vi "Test Unit Camera1.vi"() -> ()   [LabVIEW 2013]
panel:
  out "ErrorOut 2":errorcluster
  out "CameraNumber":i32
  out "Error out":i32
  out "ErrorOut":errorcluster {"code" format="%x"}
  out "Description":T1 {"GeneralCapabilities 2" format="%032b"; "GeneralCapabilities" format="%032b"; "SensorSubtypeDESC" format="%.0x"; "SensorTypeDESC" format="%.0x"}
  in  "Interface Type":u32=3
  in  "CamNumIn":i32
  in  "Handle in":u64
  out "Error":i32
  out "CameraType":T2
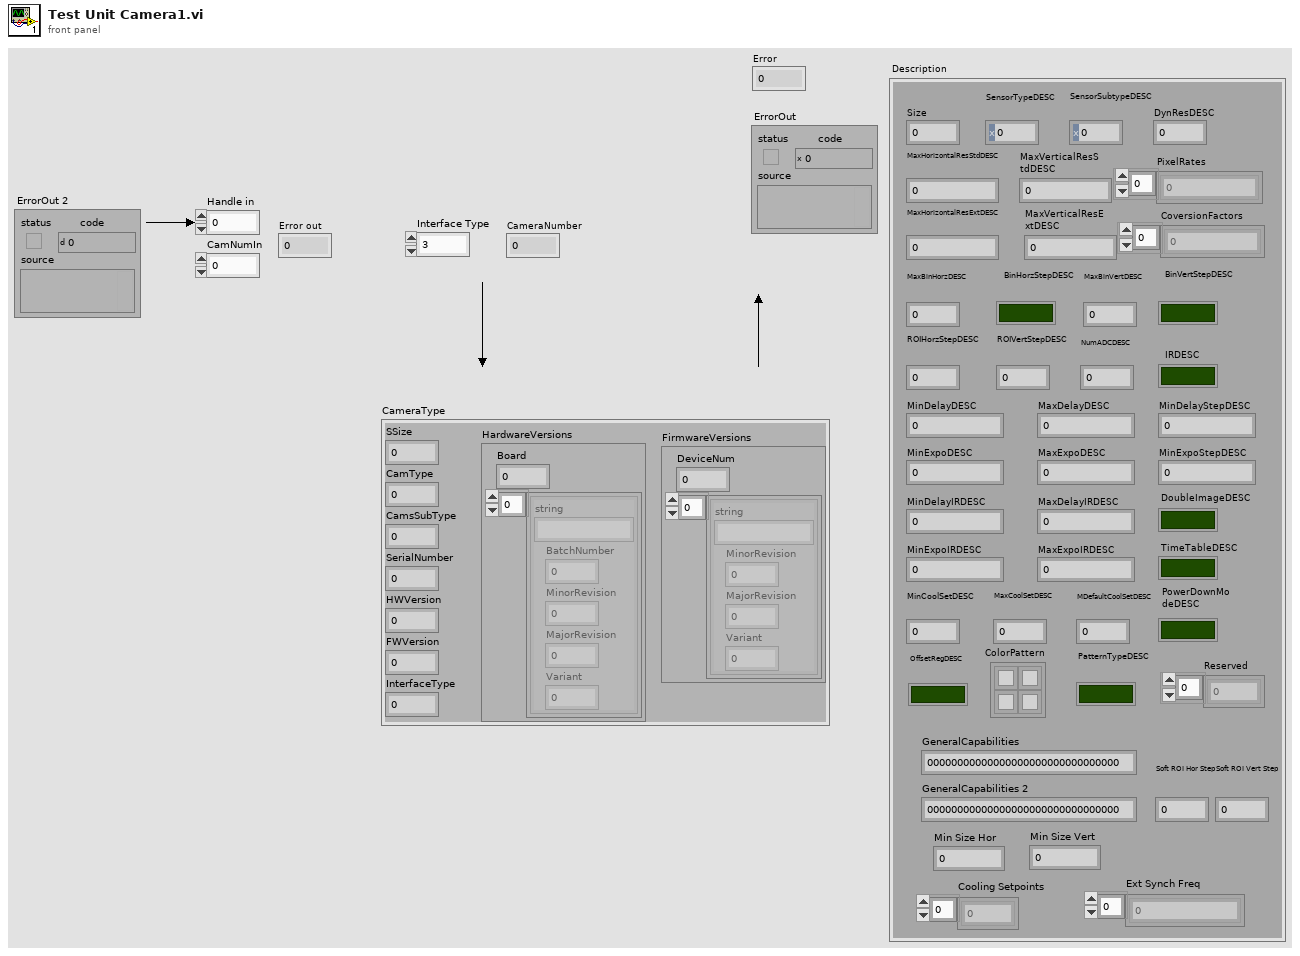
[diagram p1: front panel]
types:
  T1 = cluster{"Size":u16, "SensorTypeDESC":u16, "SensorSubtypeDESC":u16, "MaxHorizontalResStdDESC":u16, "MaxVerticalResStdDESC":u16, "MaxHorizontalResExtDESC":u16, "MaxVerticalResExtDESC":u16, "DynResDESC":u16, "MaxBinHorzDESC":u16, "BinHorzStepDESC":bool, "MaxBinVertDESC":u16, "BinVertStepDESC":bool, "ROIHorzStepDESC":u16, "ROIVertStepDESC":u16, "NumADCDESC":u16, "IRDESC":bool, "MinDelayDESC":u32, "MaxDelayDESC":u32, "MinDelayStepDESC":u32, "MinExpoDESC":u32, "MaxExpoDESC":u32, "MinExpoStepDESC":u32, "MinDelayIRDESC":u32, "MaxDelayIRDESC":u32, "MinExpoIRDESC":u32, "MaxExpoIRDESC":u32, "TimeTableDESC":bool, "DoubleImageDESC":bool, "MinCoolSetDESC":i16, "MaxCoolSetDESC":i16, "MDefaultCoolSetDESC":i16, "PowerDownModeDESC":bool, "OffsetRegDESC":bool, "ColorPattern":cluster{"UpperLeftColor":u8, "UpperRightColor":u8, "LowerLeftColor":u8, "LowerRightColor":u8}, "PatternTypeDESC":bool, "PixelRates":u32[], "CoversionFactors":u16[], "Reserved":u32[], "GeneralCapabilities":u32, "GeneralCapabilities 2":u32, "Min Size Hor":u16, "Min Size Vert":u16, "Ext Synch Freq":u32[], "Cooling Setpoints":i16[], "Soft ROI Hor Step":u16, "Soft ROI Vert Step":u16}
  T2 = cluster{"SSize":u16, "CamType":u16, "CamsSubType":u16, "SerialNumber":u32, "HWVersion":u32, "FWVersion ":u32, "InterfaceType":u16, "HardwareVersions":cluster{"Board":u16, cluster{"string":string, "BatchNumber":u16, "MinorRevision":u8, "MajorRevision":u8, "Variant":u16}[]}, "FirmwareVersions":cluster{"DeviceNum":u16, cluster{"string":string, "MinorRevision":u8, "MajorRevision":u8, "Variant":u16}[]}}
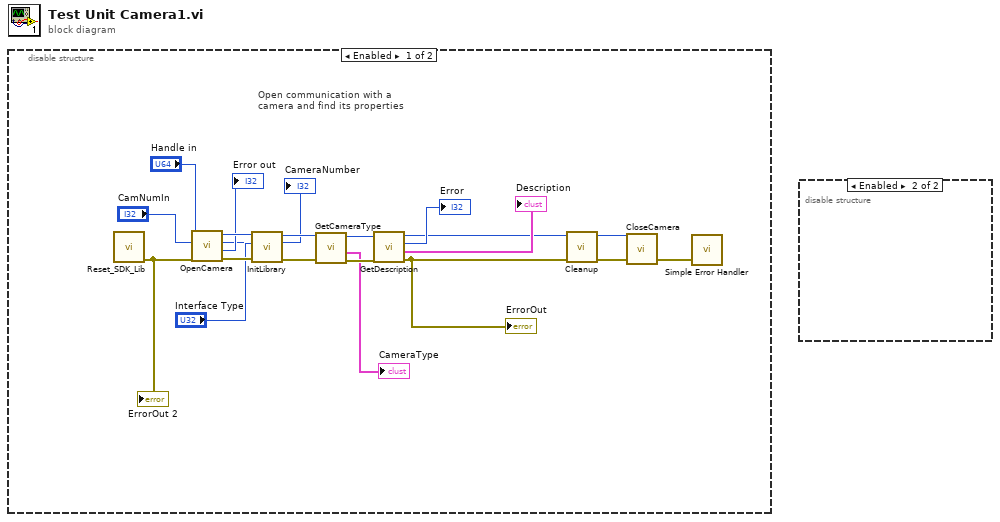
[diagram p0: block diagram]
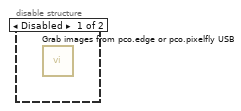
[diagram p3: hidden frame]
diagram:
  n1 = disable-structure shown="Enabled" {
    frame Enabled {
      # "Open communication with a camera and find its properties"
      n2 = call <userlib>:"Reset_SDK_Lib.vi"() -> ("ErrorOut"=w13:errorcluster)  [unwired: 11 in]
      "ErrorOut 2" <- w13
      n3 = call <userlib>:"OpenCamera.vi"("ErrorIn"=w13, "CamNumIn"="CamNumIn", "Handle in"="Handle in") -> ("ErrorOut"=w17:errorcluster, "Error out"=→"Error out":i32, "CameraNumber"=→"CameraNumber":i32, "Handle out"=w18:u64)  [unwired: 1 in]
      n4 = call <userlib>:"InitLibrary.vi"("error in (no error)"=w17, "InterfaceType"="Interface Type", "ph"=w18) -> ("error out"=w16:errorcluster, "hout"=w15:u64)  [unwired: 7 in]
      n5 = call <userlib>:"GetCameraType.vi"("ph"=w15, "error in (no error)"=w16) -> ("hout"=w20:u64, "CameraType"=→"CameraType":T2, "error out"=w19:errorcluster)  [unwired: 1 in, 1 out]
      n6 = call <userlib>:"GetDescription.vi"("ErrorIn"=w19, "ph"=w20) -> ("ErrorOut"=w1:errorcluster, "Description"=→"Description":T1, "Error"=→"Error":i32, "hout"=w2:u64)  [unwired: 2 in]
      "ErrorOut" <- w1
      n7 = call <userlib>:"Cleanup.vi"("error in (no error)"=w1, "ph"=w2) -> ("error out"=w3:errorcluster, "hout"=w4:u64)  [unwired: 8 in]
      n8 = call <userlib>:"CloseCamera.vi"("ErrorIn"=w3, "Handle in"=w4) -> ("ErrorOut"=w5:errorcluster)  [unwired: 1 in, 2 out]
      n9 = call <vilib>:"Simple Error Handler.vi"("error in (no error)"=w5) -> ()  [unwired: 4 in, 5 out]
    }
    frame Disabled {
    }
  }
  n10 = disable-structure shown="Enabled" {
    frame Disabled {
      n11 = call <userlib>:"Grab images from pco.edge or pco.pixelfly USB.vi"() -> ()  [unwired: 1 in]
    }
    frame Enabled {
    }
  }
